vi "control_camera_properties.vi"(8 "error in (no error)":errorcluster, 10 "Control Camera Properties":T1={"Packet Size"=1500, "Pixel Format"=17825797, "Gain in dB"=1.0, "Exposure Time in µs"=1500, "Stream Bytes per Second"=50000000} {"Stream Bytes per Second" min=1000000 max=124000000 step=1 format="%.0p"; "Exposure Time in µs" min=21 max=153391689 format="%#.0f"; "Gain in dB" min=0.0 max=26.0 format="%#_2g"; "Pixel Format" items=["Mono 12 Packed"=17563654, "Mono 12"=17825797, "Mono 8"=17301505]}, 11 "IMAQdx Session":T2) -> (0 "error out 2":errorcluster, 2 "output cluster":T1={"Packet Size"=1500, "Pixel Format"=17825797, "Gain in dB"=1.0, "Exposure Time in µs"=1500, "Stream Bytes per Second"=50000017} caption="Control Camera Properties" {"Stream Bytes per Second" min=1000000 max=124000000 step=100000 format="%.1p"; "Exposure Time in µs" min=21 max=153391689 format="%#.0f"; "Gain in dB" min=0.0 max=26.0 format="%#_2g"; "Pixel Format" items=["Mono 12 Packed"=17563654, "Mono 12"=17825797]}, 3 "Session Out 2":T2)   [LabVIEW 2014]
uses:
  <vilib>/userdefined/High Color/IMAQdx.ctl
  type definitions/control camera properties.ctl
  <resource>/objmgr/imaqdx.rc
panel:
  # "Bytes"
  # "Trigger"
  # "Bytes"
  # "Trigger"
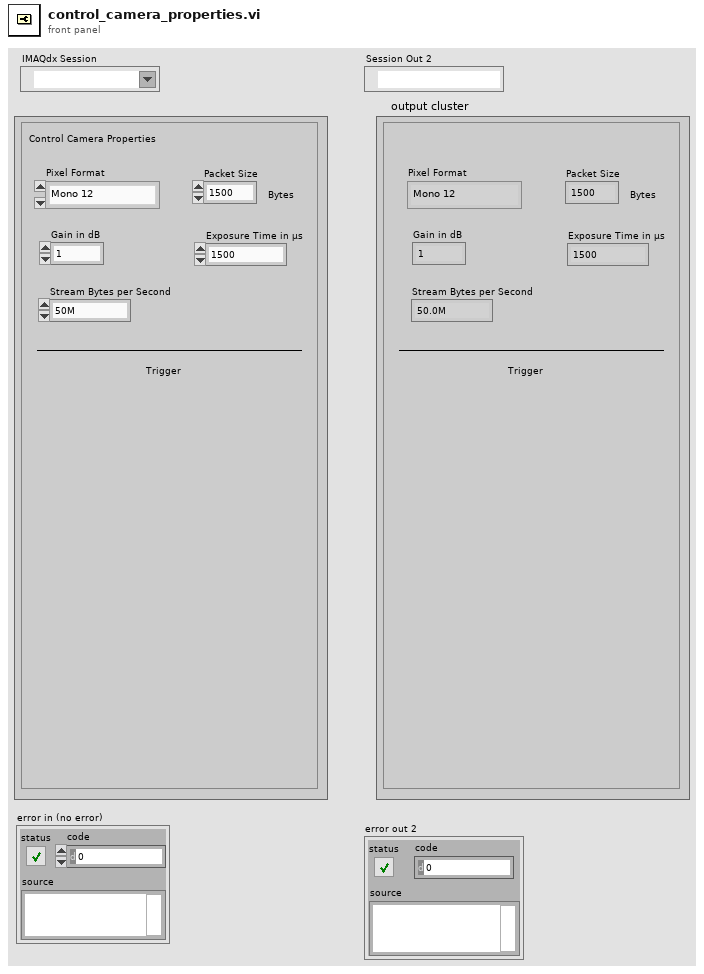
[diagram p1: front panel]
types:
  T1 = typedef "control camera properties.ctl" = cluster{"Packet Size":u32, "Pixel Format":u32, "Gain in dB":dbl, "Exposure Time in µs":u32, "Stream Bytes per Second":u32}
  T2 = typedef "IMAQdx.ctl" = refnum<k21>
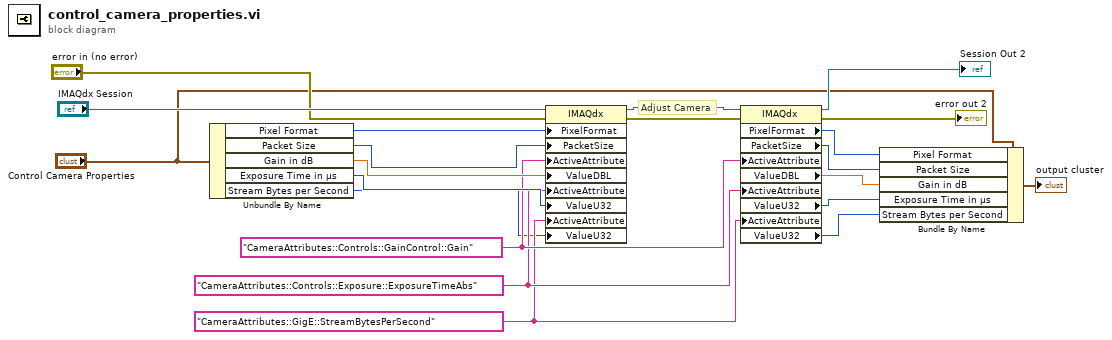
[diagram p0: block diagram]
diagram:
  w5 = "CameraAttributes::GigE::StreamBytesPerSecond"
  w13 = "CameraAttributes::Controls::Exposure::ExposureTimeAbs"
  w14 = "CameraAttributes::Controls::GainControl::Gain"
  # "Adjust Camera"
  n1 = Unbundle By Name("Control Camera Properties") -> ("Pixel Format"=w19:u32, "Packet Size"=w18:u32, "Gain in dB"=w17:dbl, "Exposure Time in µs"=w16:u32, "Stream Bytes per Second"=w4:u32)
  n2 = property class="IMAQdx"(reference="IMAQdx Session", error in="error in (no error)", "PixelFormat"=w19, "PacketSize"=w18, "ActiveAttribute"=w14, "ValueDBL"=w17, "ActiveAttribute"=w13, "ValueU32"=w16, "ActiveAttribute"=w5, "ValueU32"=w4) -> (reference out=w15:T2, error out=w8:errorcluster)
  n3 = property class="IMAQdx"(reference=w15, error in=w8, "ActiveAttribute"=w14, "ActiveAttribute"=w13, "ActiveAttribute"=w5) -> (reference out=→"Session Out 2":T2, error out=→"error out 2":errorcluster, "PixelFormat"=w12:u32, "PacketSize"=w11:u32, "ValueDBL"=w10:dbl, "ValueU32"=w9:u32, "ValueU32"=w3:u32)
  n4 = Bundle By Name(cluster="Control Camera Properties", "Pixel Format"=w12, "Packet Size"=w11, "Gain in dB"=w10, "Exposure Time in µs"=w9, "Stream Bytes per Second"=w3) -> (→"output cluster":T1)
